vi "Controller Subscriber.vi"() -> ()   [LabVIEW 2015]
uses:
  <userlib>/ROS for LabVIEW Software/ROS/Code/Console/Servers/ServerSubs/TopicDef.ctl
  <userlib>/ROS for LabVIEW Software/ROS/Code/SubVIs/_ROSDirection.ctl
panel:
  in  "Stop Button":bool
  out "String":string
  in  "Definitions":T1={"Topic"="/controller", "Type"="std_msgs/String", "Action"=enum."Subscriber", "Update (ms)"=10, "queue size"=100}
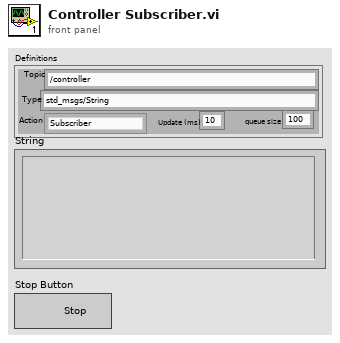
[diagram p1: front panel]
types:
  T1 = typedef "TopicDef.ctl" = cluster{"Topic":string, "Type":string, "Action":T2, "Update (ms)":u16, "queue size":u16}
  T2 = typedef "_ROSDirection.ctl" = enum16{"Node", "Publisher", "Subscriber", "ServiceClient", "ServiceProvider"}
  T3 = typedef "_ROSControl.ctl" = cluster{"topic port":u16, "Node":string, "topic":string, "type":string, "node port":u16, "error ":errorcluster, "Direction":T2, "Update (ms)":u16, "FIFO size":u16}
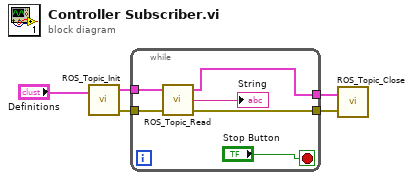
[diagram p0: block diagram]
diagram:
  n1 = call <userlib>:"ROS_Topic_Init.vi"("Definitions"="Definitions") -> ("ROS out"=w2:T3, "error out"=w1:errorcluster)  [unwired: 2 in]
  n2 = while {
    tunnel: [w10] -> w5
    tunnel: [w7] -> w4
    tunnel: w2 -> [w8]
    tunnel: w1 -> [w9]
    stop <- "Stop Button" stop-if-true
    n3 = call <userlib>:"ROS_Topic_Read.vi"("error in (no error)"=w9, "ROS in"=w8) -> ("error out"=w7:errorcluster, "Reply"=→"String":string, "ROS out"=w10:T3)  [unwired: 1 in]
  }
  n4 = call <userlib>:"ROS_Topic_Close.vi"("error in"=w4, "ROS in"=w5) -> ()  [unwired: 2 in, 1 out]
